vi "GE5565 Read-Mod-Write 32 mod.vi"(4 "value":u32 format="%.0x", 6 "inv bit mask":u32=264448 format="%.0x", 7 "address space (13: BAR2)":u16=13, 8 "error in (no error)":errorcluster, 10 "offset (0)":u32 format="%.0x", 11 "VISA resource name":refnum<visa-resource-name>) -> (0 "error out":errorcluster, 3 "VISA resource name out":refnum<visa-resource-name>)   [LabVIEW 2017, in "GE_RM_Real Time.lvlib"]
uses:
  GE_RM_Real Time.lvlib
panel:
  out "x .or. y?":u32 format="%032b"
  out "result":u32 format="%032b"
  out "inv bit mask 2":u32 format="%032b"
  out "value 2":u32 format="%032b"
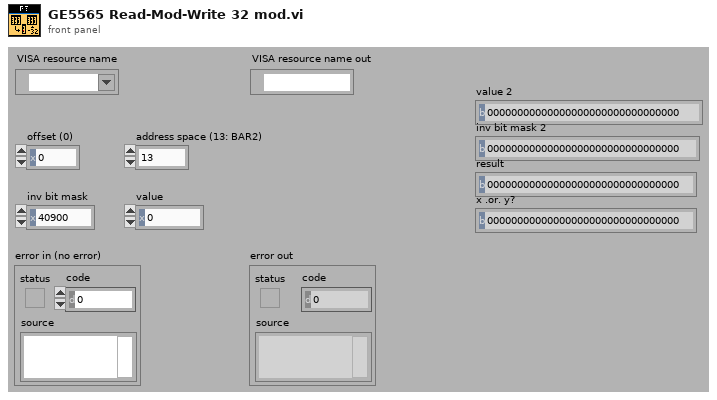
[diagram p1: front panel]
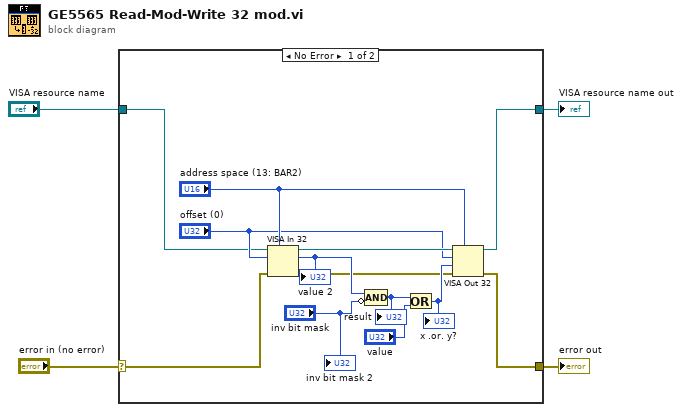
[diagram p0: block diagram]
diagram:
  n1 = case shown="No Error" "error in (no error)" {
    selector: "error in (no error)" -> [w17 w18]
    tunnel: "VISA resource name" -> [w5 w19]
    tunnel: [w6 w19] -> w2
    tunnel: [w7 w18] -> w3
    frame No Error {
      n2 = VISA In 32(7:"address space (13: BAR2)", 8:w17, 10:"offset (0)", 11:w5) -> (0:w9:errorcluster, 2:w16:u32, 3:w10:refnum<visa-resource-name>)
      "value 2" <- w16
      n3 = Compound Arithmetic op=AND(w16, invert "inv bit mask") -> (w14:u32)
      "result" <- w14
      n4 = Or(x=w14, y="value") -> (x .or. y?=w12:u32)
      "x .or. y?" <- w12
      n5 = VISA Out 32(7:"address space (13: BAR2)", 8:w9, 9:w12, 10:"offset (0)", 11:w10) -> (0:w7:errorcluster, 3:w6:refnum<visa-resource-name>)
      "inv bit mask 2" <- "inv bit mask"
    }
    frame Error {
    }
  }
  "error out" <- w3
  "VISA resource name out" <- w2
